vi "DPTest-Simulate Cal Signal.vi"(0 "Speakers":string[](array[string]), 1 "freqs":dbl[](array[numeric]), 2 "Attenuation (dB)":dbl[](array[numeric]), 3 "Acoustic system":string, 5 "ceilings":dbl[](array[numeric]), 7 "state":T1, 11 "error in (no error)":errorcluster, 12 "Nbuf":i32=10000) -> (15 "error out":errorcluster)   [LabVIEW 2020]
uses:
  Typedefs/DP-Runtime State.ctl
  epl-vi-lib/Signal Synthesis VIs/4th Generation/Classes/Gate/Gate.lvclass/Gate.ctl
  bc6414e4-3673-4db9-9987-8075f6ebf4c6.vi
  4d7382aa-da82-4a5e-b546-f30b57a76c94.vi
  epl-vi-lib/Signal Synthesis VIs/4th Generation/Common/CommonSig-Apply Ramp (2D).vi
  90a97fba-9c1e-4e2a-8569-7bbd5edfb3ea.vi
  50cf06c4-ddb6-403d-aefe-4311d7d37b60.vi
  8a331112-bbc1-4753-9b51-6dceaaeb95e8.vi
  epl-vi-lib/Signal Synthesis VIs/4th Generation/Common/CommonSig-Apply Ramp (2D).vi/00fa021d-ebe0-42e5-9c35-5538040c7da1.vi
  epl-vi-lib/Signal Synthesis VIs/4th Generation/Classes/Gate/Write Ramp (ms).vi
  epl-vi-lib/Signal Synthesis VIs/4th Generation/Classes/Gate/Write Down (ms).vi
  epl-vi-lib/Signal Synthesis VIs/4th Generation/Classes/Gate/Write Asymmetric.vi
  epl-vi-lib/Signal Synthesis VIs/4th Generation/Classes/Gate/Write Shape.vi
  epl-vi-lib/Signal Synthesis VIs/4th Generation/Classes/Gate/Write Duration (ms).vi
  epl-vi-lib/PXI DAQ VIs/AIDI/AIDI-Engine.vi
  epl-vi-lib/Signal Synthesis VIs/4th Generation/Classes/Gate/Create.vi
  epl-vi-lib/Signal Synthesis VIs/4th Generation/Classes/Gate/Apply.vi
  epl-cal-vi-lib/Common VIs/Typedefs/CAL-Globals.vi
  epl-vi-lib/PXI DAQ VIs/AODO/AODO-Engine.vi
  <vilib>/Analysis/NI_AALBase.lvlib
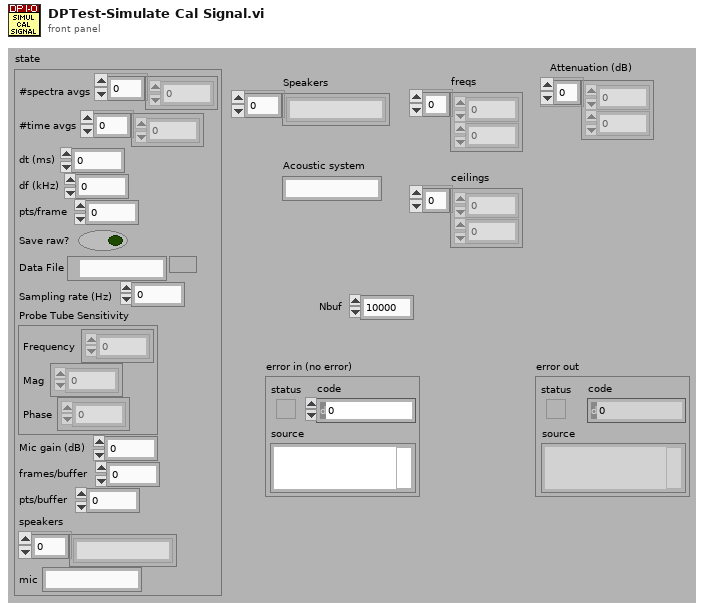
[diagram p1: front panel]
types:
  T1 = typedef "DP-Runtime State.ctl" = cluster{"#spectra avgs":i32[], "#time avgs":i32[], "dt (ms)":dbl, "df (kHz)":dbl, "pts/frame":i32, "Save raw?":bool, "Data File":path, "Sampling rate (Hz)":dbl, "Probe Tube Sensitivity":cluster{"Frequency":dbl[], "Mag":dbl[], "Phase":dbl[]}, "Mic gain (dB)":dbl, "frames/buffer":i32, "pts/buffer":i32, "speakers":string[], "mic":string}
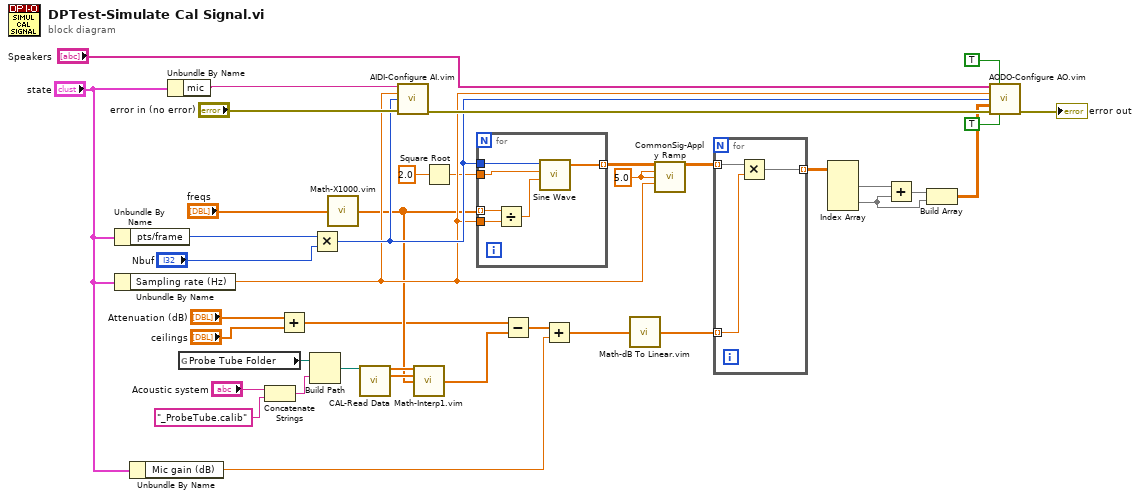
[diagram p0: block diagram]
diagram:
  w31 = 5.0 ("Ramp up (ms)")
  n1 = Unbundle By Name("state") -> ("pts/frame"=w30:i32)
  n2 = Unbundle By Name("state") -> ("Sampling rate (Hz)"=w28:dbl)
  n3 = Unbundle By Name("state") -> ("Mic gain (dB)"=w13:dbl)
  n4 = Unbundle By Name("state") -> ("mic"=w29:string)
  n5 = global read "CAL-Globals.vi" "Probe Tube Folder"() -> (w23:path)
  n6 = Concatenate Strings("Acoustic system", "_ProbeTube.calib" ("string")) -> (w24:string)
  n7 = Add(x="Attenuation (dB)", y="ceilings") -> (x+y=w16:dbl[])
  n8 = Build Path(base path=w23, name or relative path=w24) -> (appended path=w22:path)
  n9 = Multiply(x=w30, y="Nbuf") -> (x*y=w33:i32)
  n10 = call "Math-X1000.vim"("X"="freqs") -> ("1000X"=w17:dbl[])
  n11 = call "CAL-Read Data.vi"("user path"=w22) -> ("Frequency (Hz)"=w21:dbl[], "Mag"=w20:dbl[])  [unwired: 10 in, 3 out]
  n12 = call "AIDI-Configure AI.vim"("AI.Channels"=w29, "AI.Fs (Hz)"=w28, "AI.Npts"=w33, "error in (no error)"="error in (no error)") -> ("error out"=w36:errorcluster)  [unwired: 11 in]
  n13 = call "Math-Interp1.vim"("X"=w21, "Y"=w20, "U"=w17) -> ("V"=w15:dbl[])  [unwired: 12 in]
  n14 = Square Root(x=2.0) -> (sqrt(x)=w3:dbl)
  n15 = for {
    tunnel: w17 -> [w43] mode=indexing
    tunnel: w3 -> [w44]
    tunnel: w33 -> [w45]
    tunnel: w28 -> [w41]
    tunnel: [w40] -> w32 mode=indexing
    n16 = Divide(x=w43, y=w41) -> (x/y=w42:dbl)
    n17 = call <vilib>:"Sine Wave.vi"("samples"=w45, "amplitude"=w44, "frequency"=w42) -> ("sine wave"=w40:dbl[])  [unwired: 2 in, 2 out]
  }
  n18 = Subtract(x=w16, y=w15) -> (x-y=w14:dbl[])
  n19 = Add(x=w14, y=w13) -> (x+y=w11:dbl[])
  n20 = call "Math-dB To Linear.vim"("dB"=w11) -> ("linear"=w5:dbl[])
  n21 = call-poly "CommonSig-Apply Ramp.vi"("Array in"=w32, "Ramp up (ms)"=w31, "Ramp down (ms)"=w31, "Fs (Hz)"=w28) -> ("Array out"=w12:dbl[][])  [unwired: 10 in, 1 out]
  n22 = for {
    tunnel: w12 -> [w48] mode=indexing
    tunnel: w5 -> [w47] mode=indexing
    tunnel: [w46] -> w10 mode=indexing
    n23 = Multiply(x=w48, y=w47) -> (x*y=w46:dbl[])
  }
  n24 = Index Array(array=w10) -> (element #1=w9:dbl[], element #2=w7:dbl[])  [unwired: 4 in]
  n25 = Add(x=w9, y=w7) -> (x+y=w8:dbl[])
  n26 = Build Array(w8, w7) -> (w6:dbl[][])
  n27 = call "AODO-Configure AO.vim"("AO.Channels"="Speakers", "Finite"=TRUE, "AO.Fs (Hz)"=w28, "AO.Npts"=w33, "AO"=w6, "error in (no error)"=w36, "Allow regen? (F)"=TRUE) -> ("error out"=→"error out":errorcluster)  [unwired: 8 in]
